vi "determine_motshutter_column.vi"(1 "MOT Shutter\nOpening Time (s)":dbl=0.05, 2 "Flash Column":i32=11, 3 "PulseBlaster Array of Arrays In":T1(array[cluster])=[{"Data Field"=0, "Delay"=0.005, "OP code"=8, "Output Bits"=[FALSE, TRUE, FALSE, FALSE, FALSE, FALSE, FALSE, FALSE, FALSE, FALSE, FALSE, FALSE, TRUE, FALSE, FALSE, FALSE, FALSE, FALSE, FALSE, FALSE, FALSE, FALSE, FALSE, FALSE], "String"="cool mot coils"}, {"Data Field"=300, "Delay"=0.000999, "OP code"=2, "Output Bits"=[TRUE, TRUE, TRUE, TRUE, FALSE, FALSE, TRUE, FALSE, FALSE, TRUE, FALSE, FALSE, TRUE, TRUE, FALSE, TRUE, TRUE, FALSE, FALSE, FALSE, FALSE, FALSE, FALSE, FALSE], "String"="mot load loop"}, {"Data Field"=1, "Delay"=1e-06, "OP code"=3, "Output Bits"=[TRUE, TRUE, TRUE, TRUE, FALSE, FALSE, TRUE, FALSE, FALSE, TRUE, FALSE, FALSE, TRUE, TRUE, FALSE, TRUE, TRUE, FALSE, FALSE, FALSE, FALSE, FALSE, FALSE, FALSE, FALSE], "String"=""}, {"Data Field"=0, "Delay"=0.001, "OP code"=0, "Output Bits"=[TRUE, TRUE, TRUE, TRUE, FALSE, FALSE, TRUE, FALSE, FALSE, TRUE, FALSE, FALSE, TRUE, TRUE, FALSE, TRUE, TRUE, FALSE, FALSE, FALSE, FALSE, FALSE, FALSE, FALSE], "String"=""}, {"Data Field"=2, "Delay"=0.000999, "OP code"=2, "Output Bits"=[TRUE, TRUE, TRUE, TRUE, FALSE, FALSE, TRUE, FALSE, FALSE, TRUE, FALSE, FALSE, TRUE, TRUE, FALSE, TRUE, TRUE, FALSE, FALSE, FALSE, FALSE, FALSE, FALSE, FALSE], "String"="mot decay loop"}, {"Data Field"=4, "Delay"=1e-06, "OP code"=3, "Output Bits"=[TRUE, TRUE, TRUE, TRUE, FALSE, FALSE, TRUE, FALSE, FALSE, TRUE, FALSE, FALSE, TRUE, TRUE, FALSE, TRUE, TRUE, FALSE, FALSE, FALSE, FALSE, FALSE, FALSE, FALSE], "String"=""}, {"Data Field"=0, "Delay"=0.04, "OP code"=0, "Output Bits"=[TRUE, TRUE, TRUE, TRUE, FALSE, FALSE, TRUE, FALSE, FALSE, TRUE, FALSE, FALSE, TRUE, TRUE, FALSE, TRUE, TRUE, FALSE, FALSE, FALSE, FALSE, FALSE, FALSE, FALSE], "String"=""}, {"Data Field"=0, "Delay"=0.00865, "OP code"=0, "Output Bits"=[TRUE, TRUE, TRUE, TRUE, FALSE, FALSE, TRUE, FALSE, FALSE, TRUE, FALSE, FALSE, TRUE, TRUE, FALSE, TRUE, TRUE, FALSE, FALSE, FALSE, FALSE, FALSE, FALSE, FALSE], "String"=""}, {"Data Field"=0, "Delay"=0.004, "OP code"=0, "Output Bits"=[TRUE, TRUE, FALSE, TRUE, FALSE, FALSE, TRUE, FALSE, FALSE, TRUE, FALSE, FALSE, TRUE, TRUE, FALSE, TRUE, TRUE, FALSE, FALSE, FALSE, FALSE, FALSE, FALSE, FALSE], "String"=""}, {"Data Field"=0, "Delay"=0.0045, "OP code"=0, "Output Bits"=[TRUE, TRUE, FALSE, TRUE, FALSE, FALSE, TRUE, FALSE, FALSE, TRUE, FALSE, FALSE, TRUE, FALSE, FALSE, FALSE, TRUE, FALSE, FALSE, FALSE, FALSE, FALSE, FALSE, FALSE], "String"="Blue MOT Cooling Time"}, {"Data Field"=0, "Delay"=0.05, "OP code"=0, "Output Bits"=[FALSE, TRUE, FALSE, FALSE, FALSE, FALSE, FALSE, FALSE, FALSE, TRUE, TRUE, FALSE, TRUE, FALSE, FALSE, FALSE, FALSE, FALSE, FALSE, FALSE, FALSE, FALSE, FALSE, FALSE], "String"="Red MOT Cooling Time =="}, {"Data Field"=0, "Delay"=0.01, "OP code"=0, "Output Bits"=[FALSE, TRUE, FALSE, FALSE, FALSE, FALSE, FALSE, FALSE, FALSE, FALSE, FALSE, FALSE, FALSE, FALSE, FALSE, FALSE, FALSE, FALSE, FALSE, FALSE, FALSE, FALSE, FALSE, FALSE], "String"="PAS Beam with RED MOT            DELAY TIME BEFORE INTERAC"}, {"Data Field"=0, "Delay"=0.005, "OP code"=0, "Output Bits"=[FALSE, TRUE, FALSE, FALSE, FALSE, FALSE, FALSE, FALSE, FALSE, FALSE, FALSE, FALSE, FALSE, FALSE, FALSE, FALSE, TRUE, FALSE, FALSE, FALSE, FALSE, FALSE, FALSE, FALSE], "String"="image 12 delay (150n=90ndelay) INTERAC TIME"}, {"Data Field"=0, "Delay"=5e-05, "OP code"=0, "Output Bits"=[FALSE, TRUE, FALSE, FALSE, FALSE, FALSE, FALSE, FALSE, FALSE, FALSE, FALSE, FALSE, FALSE, FALSE, FALSE, FALSE, TRUE, TRUE, FALSE, FALSE, FALSE, FALSE, FALSE, FALSE], "String"="image beam on"}, {"Data Field"=0, "Delay"=0.0002, "OP code"=0, "Output Bits"=[FALSE, FALSE, FALSE, FALSE, FALSE, TRUE, FALSE, FALSE, FALSE, FALSE, FALSE, FALSE, FALSE, FALSE, FALSE, FALSE, TRUE, TRUE, FALSE, FALSE, FALSE, FALSE, FALSE, FALSE], "String"="camera minimum exposure time"}, {"Data Field"=0, "Delay"=0.07, "OP code"=0, "Output Bits"=[FALSE, FALSE, FALSE, FALSE, FALSE, FALSE, FALSE, FALSE, FALSE, FALSE, FALSE, FALSE, FALSE, FALSE, FALSE, FALSE, FALSE, TRUE, FALSE, FALSE, FALSE, FALSE, FALSE, FALSE], "String"="PixelFly Readout 1"}, {"Data Field"=0, "Delay"=0.005, "OP code"=0, "Output Bits"=[FALSE, FALSE, FALSE, FALSE, FALSE, FALSE, FALSE, FALSE, FALSE, FALSE, FALSE, FALSE, FALSE, FALSE, FALSE, FALSE, TRUE, TRUE, FALSE, FALSE, FALSE, FALSE, FALSE, FALSE], "String"="shutter opening time"}, {"Data Field"=0, "Delay"=0.0002, "OP code"=0, "Output Bits"=[FALSE, FALSE, FALSE, FALSE, FALSE, TRUE, FALSE, FALSE, FALSE, FALSE, FALSE, FALSE, FALSE, FALSE, FALSE, FALSE, TRUE, TRUE, FALSE, FALSE, FALSE, FALSE, FALSE, FALSE], "String"="Pixelfly exposure 2"}, {"Data Field"=0, "Delay"=0.07, "OP code"=0, "Output Bits"=[FALSE, FALSE, FALSE, FALSE, FALSE, FALSE, FALSE, FALSE, FALSE, FALSE, FALSE, FALSE, FALSE, FALSE, FALSE, FALSE, FALSE, FALSE, FALSE, FALSE, FALSE, FALSE, FALSE, FALSE], "String"="PixelFly readout 2"}, {"Data Field"=0, "Delay"=0.001, "OP code"=6, "Output Bits"=[FALSE, TRUE, TRUE, TRUE, FALSE, FALSE, FALSE, FALSE, FALSE, FALSE, FALSE, FALSE, TRUE, TRUE, FALSE, TRUE, FALSE, FALSE, FALSE, FALSE, FALSE, FALSE, FALSE, FALSE], "String"=""}] {"OP code" items=["Continue", "Stop", "Loop", "End Loop", "Jump", "Return", "Go To", "Long Delay", "Wait"]; "Delay" format="%.3p"}) -> (0 "Column at which\nto open MOT shutter":i32=10)   [LabVIEW 2013]
panel:
  # "This VI sums up the times from columns before the\nMOT flash column and compares this time to the MOT\nshutter opening time (e.g. 50 ms).  When it exceeds\nthe MOT shutter opening time, the current column is\nreturned as the column where the MOT shutter must\nbegin opening."
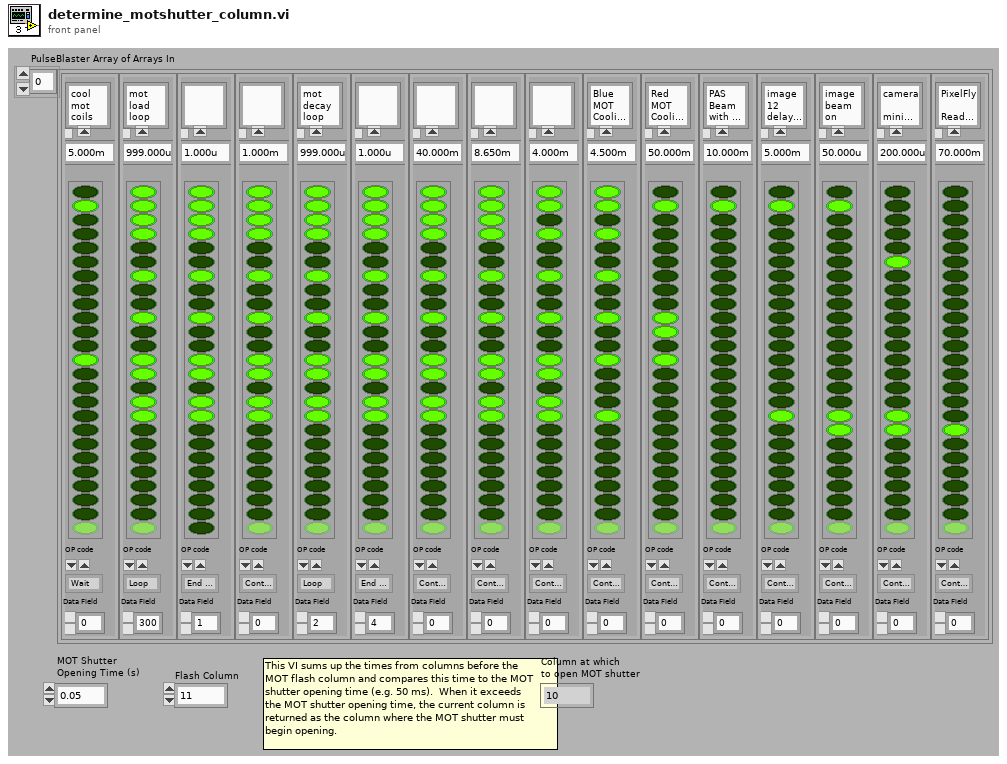
[diagram p1: front panel]
types:
  T1 = cluster{"Data Field":u32, "Delay":dbl, "OP code":u8, "Output Bits":bool[], "String":string}[]
  T2 = cluster{"Data Field":u32, "Delay":dbl, "OP code":u8, "Output Bits":bool[], "String":string}
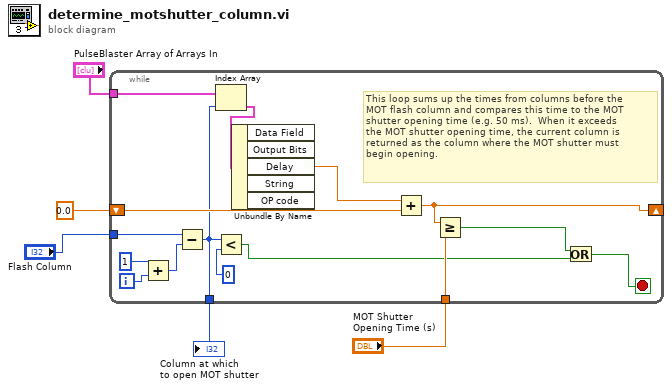
[diagram p0: block diagram]
diagram:
  n1 = while {
    tunnel: "Flash Column" -> [w17]
    tunnel: "PulseBlaster Array of Arrays In" -> [w16]
    shift-right: [w13] -> _
    shift-left: 0.0 -> [w14]
    tunnel: "MOT Shutter\nOpening Time (s)" -> [w12]
    tunnel: [w7] -> w1
    i -> [w20]
    stop <- w8 stop-if-true
    # "This loop sums up the times from columns before the\nMOT flash column and compares this time to the MOT\nshutter opening time (e.g. 50 ms).  When it exceeds\nthe MOT shutter opening time, the current column is\nreturned as the column where the MOT shutter must\nbegin opening."
    n2 = Add(x=1, y=w20) -> (x+y=w18:i32)
    n3 = Subtract(x=w17, y=w18) -> (x-y=w7:i32)
    n4 = Index Array(array=w16, index=w7) -> (element=w15:T2)
    n5 = Less?(x=w7, y=0) -> (x < y?=w10:bool)
    n6 = Unbundle By Name(w15) -> ("Delay"=w6:dbl)  [unwired: 4 out]
    n7 = Add(x=w6, y=w14) -> (x+y=w13:dbl)
    n8 = Greater Or Equal?(x=w13, y=w12) -> (x >= y?=w9:bool)
    n9 = Or(x=w9, y=w10) -> (x .or. y?=w8:bool)
  }
  "Column at which\nto open MOT shutter" <- w1
